vi "SL_WriteData.vi"(11 "Tag":T1) -> ()   [LabVIEW 2019]
uses:
  SL_Control.ctl
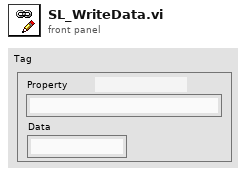
[diagram p1: front panel]
types:
  T1 = typedef "SL_Control.ctl" = cluster{"Property":string, "Type":string, "Data":string}
  T2 = cluster{"timestamp":string, "value":cluster{"type":string, "value":string}}
  T3 = enum16{"GET", "PUT", "POST", "MultiPOST", "DELETE"}
  T4 = cluster{"Name":string, "BaseURL":string, "AppKey":string, "Headers":string[], "Timeout":i32}
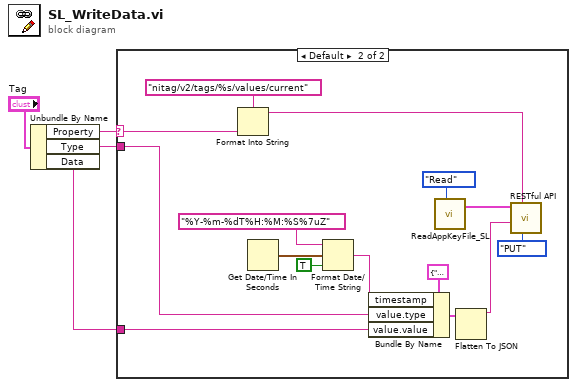
[diagram p0: block diagram]
diagram:
  n1 = Unbundle By Name("Tag") -> ("Property"=w4:string, "Type"=w2:string, "Data"=w1:string)
  n2 = case shown="Default" w4 {
    selector: w4 -> [_ w9]
    tunnel: w2 -> [_ w7]
    tunnel: w1 -> [_ w5]
    frame "" {
    }
    frame Default {
      n3 = Format Into String(format string="nitag/v2/tags/%s/values/current" ("url"), w9) -> (resulting string=w8:string)  [unwired: 2 in, 1 out]
      n4 = Get Date/Time In Seconds() -> (seconds since 1Jan1904=w14:timestamp)
      n5 = Format Date/Time String(time format string (%c)="%Y-%m-%dT%H:%M:%S%7uZ", seconds (now)=w14, UTC format=TRUE) -> (date/time string=w16:string)
      n6 = Bundle By Name(cluster=T2 {"timestamp"="", "value"={"type"="", "value"=""}}, "timestamp"=w16, "value.type"=w7, "value.value"=w5) -> (w12:T2)
      n7 = call "ReadAppKeyFile_SL.vi"("Task"=enum16{"Read", "Write"}."Read") -> ("Device Out"=w6:T4)  [unwired: 8 in, 2 out]
      n8 = Flatten To JSON(anything=w12) -> (JSON string=w10:string)  [unwired: 2 in, 1 out]
      n9 = call "RESTful API.vi"("Method"=T3."PUT", "url"=w8, "JSON"=w10, "Device In"=w6) -> ()  [unwired: 5 in, 3 out]
    }
  }
